vi "PhotonVision_CameraProcess.vi"(9 "Roll, Pitch, Yaw":T5, 10 "TRANSLATION3D":T2={"X"=-0.334, "Y"=0.125, "Z"=-0.22} {"Z" format="%14.3f"; "Y" format="%14.3f"; "X" format="%14.3f"}, 11 "CameraName":string="GENERAL_WEBCAM") -> (0 "out CameraToTarget_Pose3d":T1={"Translation3d"={"X"=0.0, "Y"=0.0, "Z"=0.0}, "Rotation3d"={"Q_quaternion"={"R"=1.0, "V"=[0.0, 0.0, 0.0]}}} {"Translation3d"."Z" format="%14.3f"; "Translation3d"."Y" format="%14.3f"; "Translation3d"."X" format="%14.3f"}, 1 "out RobotPose":T6 {"ROTATION"."SIN" format="%13.4f"; "ROTATION"."COS" format="%13.4f"; "ROTATION"."VALUE" format="%13.4f"; "TRANSLATION"."Y" format="%14.3f"; "TRANSLATION"."X" format="%14.3f"}, 2 "Have Multi-tag":bool, 3 "CameraName":string="GENERAL_WEBCAM", 5 "Pose Ambiguity":dbl)   [LabVIEW 2023]
uses:
  <vilib>/Rock Robotics/WPI/ThirdParty/PhotonVisionLib/PhotonVisionLib.lvlib
  <vilib>/Rock Robotics/WPI/ThirdParty/JAS_Junk/TrajLib/Trajectory_Library.lvlib
  <vilib>/Rock Robotics/Network Tables/NT Write Numeric Array.vi
  <vilib>/Rock Robotics/WPI/ThirdParty/JAS_Junk/TrajLib/TypeDef/TRANSLATION3D.ctl
  <vilib>/Rock Robotics/WPI/ThirdParty/JAS_Junk/TrajLib/TypeDef/QUATERNION.ctl
  <vilib>/Rock Robotics/WPI/ThirdParty/JAS_Junk/TrajLib/TypeDef/ROTATION3D.ctl
  <vilib>/Rock Robotics/WPI/ThirdParty/JAS_Junk/TrajLib/TypeDef/POSE3D.ctl
  <vilib>/Rock Robotics/Network Tables/NT Write Integer Array.vi
  <vilib>/Rock Robotics/Network Tables/NT Write Boolean.vi
  <vilib>/Rock Robotics/Network Tables/NT Write Integer.vi
  <vilib>/Rock Robotics/WPI/ThirdParty/JAS_Junk/TrajLib/VI/AprilTagFieldLayout_New2025.vi
  <vilib>/Rock Robotics/WPI/ThirdParty/JAS_Junk/TrajLib/TypeDef/TRANSLATION2D.ctl
  <vilib>/Rock Robotics/WPI/ThirdParty/JAS_Junk/TrajLib/TypeDef/ROTATION2D.ctl
  <vilib>/Rock Robotics/WPI/ThirdParty/JAS_Junk/TrajLib/TypeDef/POSE2D.ctl
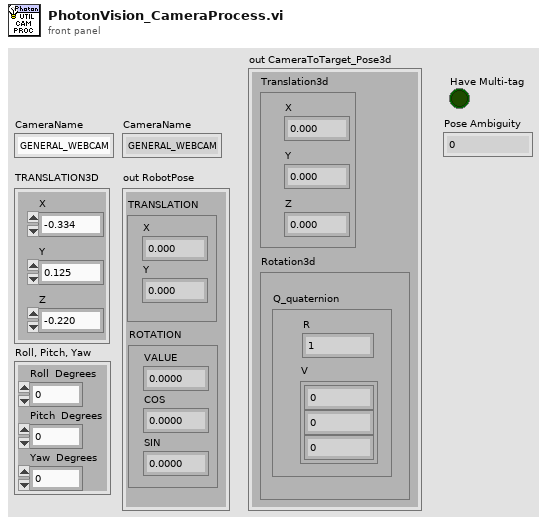
[diagram p1: front panel]
types:
  T1 = typedef "Trajectory_Library.lvlib/POSE3D.ctl" = cluster{"Translation3d":T2, "Rotation3d":T3}
  T2 = typedef "Trajectory_Library.lvlib/TRANSLATION3D.ctl" = cluster{"X":dbl, "Y":dbl, "Z":dbl}
  T3 = typedef "Trajectory_Library.lvlib/ROTATION3D.ctl" = cluster{"Q_quaternion":T4}
  T4 = typedef "Trajectory_Library.lvlib/QUATERNION.ctl" = cluster{"R":dbl, "V":dbl[]}
  T5 = cluster{"Roll  Degrees":dbl, "Pitch  Degrees":dbl, "Yaw  Degrees":dbl}
  T6 = typedef "Trajectory_Library.lvlib/POSE2D.ctl" = cluster{"TRANSLATION":T7, "ROTATION":T8}
  T7 = typedef "Trajectory_Library.lvlib/TRANSLATION2D.ctl" = cluster{"X":dbl, "Y":dbl}
  T8 = typedef "Trajectory_Library.lvlib/ROTATION2D.ctl" = cluster{"VALUE":dbl, "COS":dbl, "SIN":dbl}
  T9 = typedef "PhotonVisionLib.lvlib/PhotonPipelineResultType.ctl" = cluster{"TargetCount":i32, "Latency_MilliSec":dbl, "Targets":T10[], "TimeStampSec":dbl, "PhotonMultiTargetPNPResult":T13}
  T10 = typedef "PhotonVisionLib.lvlib/PhotonTrackedTargetType.ctl" = cluster{"Yaw":dbl, "Pitch":dbl, "Area":dbl, "Skew":dbl, "MinAreaRectCorners":T11[], "BestCameraToTarget":T12, "FiiducialId":i32, "AltCameraToTarget":T12, "PoseAmbiguity":dbl, "DetectedCorners":T11[]}
  T11 = typedef "PhotonVisionLib.lvlib/TargetCornerType.ctl" = cluster{"X":dbl, "Y":dbl}
  T12 = typedef "Trajectory_Library.lvlib/TRANSFORM3D.ctl" = cluster{"TRANSLATION3D":T2, "ROTATION3D":T3, "XF":bool}
  T13 = typedef "PhotonVisionLib.lvlib/PhotonMultiTargetPNPResultType.ctl" = cluster{"PhotonPNPResult":T14, "FiducialIDsUsed":i16[]}
  T14 = typedef "PhotonVisionLib.lvlib/PhotonPNPResultType.ctl" = cluster{"IsPresent":bool, "bestReprojErr":dbl, "altReprojErr":dbl, "ambiguity":dbl, "Best":T12, "Alt":T12}
  T15 = typedef "Trajectory_Library.lvlib/AprilTagFieldLayout.ctl" = cluster{"AprilTagMap":map{i32, T16}, "FieldLength":dbl, "FieldWidth":dbl, "OriginPosition ":T17, "OriginPose3d":T1}
  T16 = typedef "Trajectory_Library.lvlib/AprilTag.ctl" = cluster{"ID":i32, "POSE3D":T1}
  T17 = typedef "Trajectory_Library.lvlib/AprilTagFieldLayoutOrignPosition_ENUM.ctl" = enum16{"kBlueAllianceWallRightSide,", "kRedAllianceWallRightSide,"}
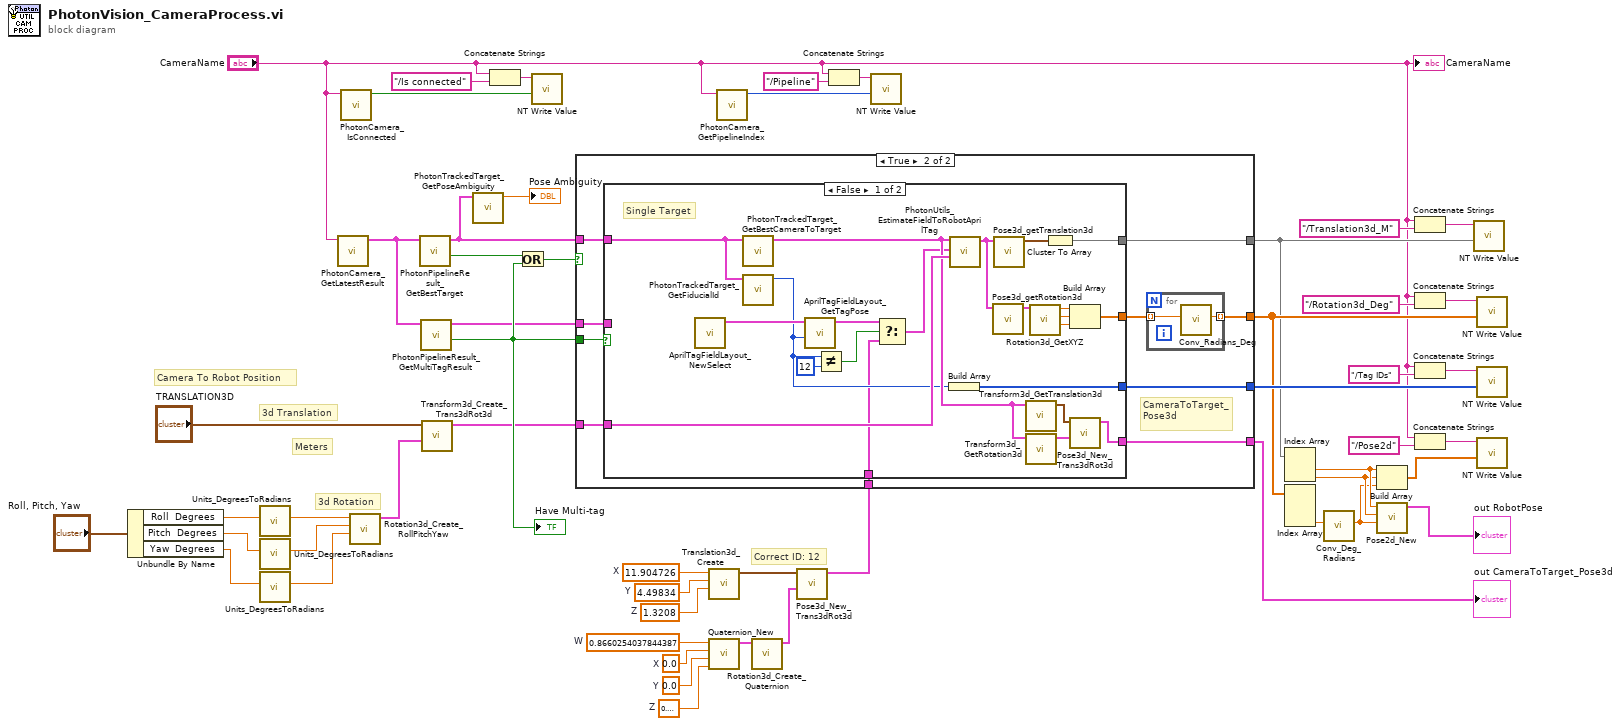
[diagram p0: block diagram]
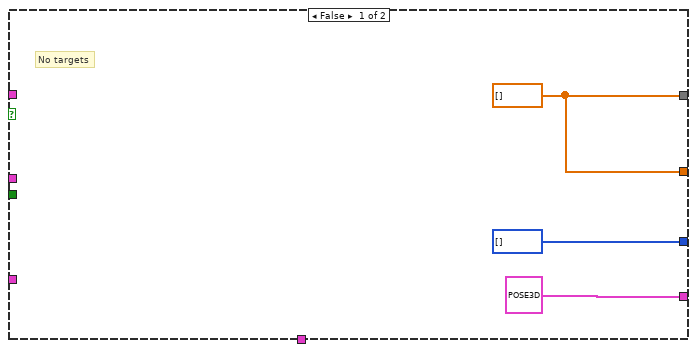
[diagram p2: hidden frame]
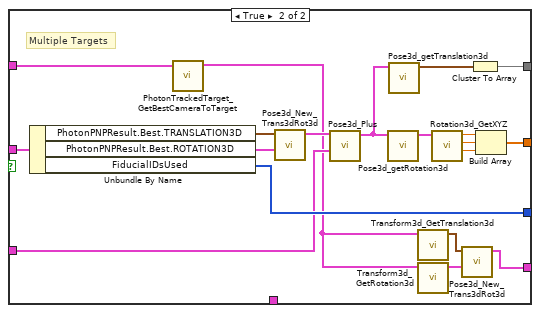
[diagram p3: hidden frame]
diagram:
  w3 = 11.904726  # X
  w4 = 4.49834  # Y
  w5 = 1.3208  # Z
  w2 = 0.8660254037844387  # W
  w6 = 0.0  # X
  w7 = 0.0  # Y
  w8 = 0.49999999999999994  # Z
  # "Correct ID: 12"
  # "Meters"
  # "Camera To Robot Position"
  # "3d Rotation"
  # "3d Translation"
  n1 = Unbundle By Name("Roll, Pitch, Yaw") -> ("Roll  Degrees"=w19:dbl, "Pitch  Degrees"=w18:dbl, "Yaw  Degrees"=w17:dbl)
  n2 = call <vilib>:"Units_DegreesToRadians.vi"("Degrees"=w19) -> ("Radians"=w46:dbl)  [unwired: 10 in]
  n3 = call <vilib>:"Units_DegreesToRadians.vi"("Degrees"=w18) -> ("Radians"=w45:dbl)  [unwired: 10 in]
  n4 = call <vilib>:"Units_DegreesToRadians.vi"("Degrees"=w17) -> ("Radians"=w44:dbl)  [unwired: 10 in]
  n5 = call <vilib>:"PhotonCamera_GetLatestResult.vi"("CameraName"="CameraName") -> ("PipelineResult"=w52:T9)  [unwired: 7 in, 3 out]
  n6 = call <vilib>:"PhotonCamera_IsConnected.vi"("CameraName"="CameraName") -> ("IsConnected"=w53:bool)  [unwired: 9 in, 1 out]
  n7 = call <vilib>:"Rotation3d_Create_RollPitchYaw.vi"("Yaw"=w44, "Pitch"=w45, "Roll"=w46) -> ("Rotation3d"=w47:T3)  [unwired: 8 in]
  n8 = call <vilib>:"PhotonPipelineResult_GetBestTarget.vi"("PhotonPipelineResult"=w52) -> ("TargetFound"=w51:bool, "PhotonTrackedTarget"=w13:T10)  [unwired: 9 in]
  n9 = call <vilib>:"PhotonPipelineResult_GetMultiTagResult.vi"("PhotonPipelineResult"=w52) -> ("Is Present"=w49:bool, "PhotonMultiTargetPNPResult"=w48:T13)  [unwired: 9 in]
  "Have Multi-tag" <- w49
  n10 = call <vilib>:"Transform3d_Create_Trans3dRot3d.vi"("Rotation3d"=w47, "Translation3d"="TRANSLATION3D") -> ("Transform3d"=w43:T12)  [unwired: 9 in]
  n11 = call <vilib>:"PhotonTrackedTarget_GetPoseAmbiguity.vi"("TrackedTarget"=w13) -> ("Pose Ambiguity"=→"Pose Ambiguity":dbl)  [unwired: 10 in]
  n12 = Concatenate Strings("CameraName", "/Is connected" ("name")) -> (w40:string)
  n13 = Or(x=w51, y=w49) -> (x .or. y?=w50:bool)
  n14 = call-poly <vilib>:"NT Write Value.vi"("value"=w53, "name"=w40) -> ()  [unwired: 9 in, 1 out]
  n15 = call <vilib>:"Translation3d_Create.vi"("Z"=w5, "Y"=w4, "X"=w3) -> ("TRANSLATION3D"=w11:T2)  [unwired: 8 in]
  n16 = call <vilib>:"Quaternion_New.vi"("Z"=w8, "Y"=w7, "X"=w6, "W"=w2) -> ("out Quaternion"=w9:T4)  [unwired: 7 in]
  n17 = call <vilib>:"PhotonCamera_GetPipelineIndex.vi"("CameraName"="CameraName") -> ("PipelineIndex"=w25:i32)  [unwired: 9 in, 1 out]
  n18 = call <vilib>:"Rotation3d_Create_Quaternion.vi"("Quaternion"=w9) -> ("Rotation3d"=w10:T3)  [unwired: 10 in]
  n19 = call <vilib>:"Pose3d_New_Trans3dRot3d.vi"("Rotation3d"=w10, "Translation3d"=w11) -> ("outPose3d"=w1:T1)  [unwired: 9 in]
  n20 = case shown="True" w50 {
    tunnel: w49 -> [_ w66]
    tunnel: w13 -> [_ w65]
    tunnel: w48 -> [_ w64]
    tunnel: w43 -> [_ w63]
    tunnel: [w56 w62] -> w29
    tunnel: [w56 w59] -> w31
    tunnel: [i16[] [] ("FiducialIDsUsed") w61] -> w42
    tunnel: [T1 {"Translation3d"={"X"=0.0, "Y"=0.0, "Z"=0.0}, "Rotation3d"={"Q_quaternion"={"R"=1.0, "V"=[0.0, 0.0, 0.0]}}} ("outPose3d") w58] -> w14
    tunnel: w1 -> [_ w57]
    frame False {
      w56 = dbl[] [] ("out Translation3d")
      # "No targets"
    }
    frame True {
      # "CameraToTarget_Pose3d"
      n21 = case shown="False" w66 {
        tunnel: w65 -> [w90 w95]
        tunnel: w64 -> [_ w109]
        tunnel: w63 -> [w88 w102]
        tunnel: [w81 w98] -> w62
        tunnel: [w80 w105] -> w61
        tunnel: [w79 w97] -> w60
        tunnel: [w75 w91] -> w58
        tunnel: w57 -> [w69 _]
        frame False {
          # "Single Target"
          n22 = call-poly <vilib>:"AprilTagFieldLayout_NewSelect.vi"() -> ("AprilTagFieldLayout"=w89:T15)  [unwired: 11 in]
          n23 = call <vilib>:"PhotonTrackedTarget_GetBestCameraToTarget.vi"("TrackedTarget"=w90) -> ("BestCameraToTarget"=w76:T12)  [unwired: 9 in, 1 out]
          n24 = call <vilib>:"PhotonTrackedTarget_GetFiducialId.vi"("TrackedTarget"=w90) -> ("Fiducial Id"=w74:i32)  [unwired: 10 in]
          n25 = call <vilib>:"AprilTagFieldLayout_GetTagPose.vi"("TagId"=w74, "AprilTagFieldLayout"=w89) -> ("TagPose3d"=w71:T1)  [unwired: 8 in, 1 out]
          n26 = Not Equal?(x=w74, y=12) -> (x != y?=w72:bool)
          n27 = Select(t=w71, s=w72, f=w69) -> (s? t:f=w70:T1)
          n28 = Build Array(w74) -> (w80:i32[])
          n29 = call <vilib>:"PhotonUtils_EstimateFieldToRobotAprilTag.vi"("CameraToRobotTransform3d"=w88, "FieldRelativeTagPose3d"=w70, "CameraToTargetTransform3d"=w76) -> ("FieldToRpbotPose3d"=w87:T1)  [unwired: 8 in]
          n30 = call <vilib>:"Pose3d_getRotation3d.vi"("in Pose3d"=w87) -> ("out Rotation3d"=w86:T3)  [unwired: 10 in]
          n31 = call <vilib>:"Pose3d_getTranslation3d.vi"("in Pose3d"=w87) -> ("out Translation3d"=w82:T2)  [unwired: 10 in]
          n32 = call <vilib>:"Transform3d_GetTranslation3d.vi"("in Transform3d"=w76) -> ("Translation3d"=w78:T2)  [unwired: 10 in]
          n33 = call <vilib>:"Transform3d_GetRotation3d.vi"("in Transform3d"=w76) -> ("Rotation3d"=w77:T3)  [unwired: 10 in]
          n34 = call <vilib>:"Rotation3d_GetXYZ.vi"("in Rotation3d"=w86) -> ("Z"=w83:dbl, "Y"=w84:dbl, "X"=w85:dbl)  [unwired: 8 in]
          n35 = Cluster To Array(cluster=w82) -> (array=w81:dbl[])
          n36 = Build Array(w85, w84, w83) -> (w79:dbl[])
          n37 = call <vilib>:"Pose3d_New_Trans3dRot3d.vi"("Rotation3d"=w77, "Translation3d"=w78) -> ("outPose3d"=w75:T1)  [unwired: 9 in]
        }
        frame True {
          # "Multiple Targets"
          n38 = Unbundle By Name(w109) -> ("PhotonPNPResult.Best.TRANSLATION3D"=w104:T2, "PhotonPNPResult.Best.ROTATION3D"=w103:T3, "FiducialIDsUsed"=w105:i16[])
          n39 = call <vilib>:"PhotonTrackedTarget_GetBestCameraToTarget.vi"("TrackedTarget"=w95) -> ("BestCameraToTarget"=w92:T12)  [unwired: 9 in, 1 out]
          n40 = call <vilib>:"Pose3d_New_Trans3dRot3d.vi"("Rotation3d"=w103, "Translation3d"=w104) -> ("outPose3d"=w96:T1)  [unwired: 9 in]
          n41 = call <vilib>:"Pose3d_Plus.vi"("other Transform3d"=w102, "in Pose3d"=w96) -> ("out Pose3d"=w100:T1)  [unwired: 9 in]
          n42 = call <vilib>:"Pose3d_getRotation3d.vi"("in Pose3d"=w100) -> ("out Rotation3d"=w101:T3)  [unwired: 10 in]
          n43 = call <vilib>:"Pose3d_getTranslation3d.vi"("in Pose3d"=w100) -> ("out Translation3d"=w99:T2)  [unwired: 10 in]
          n44 = call <vilib>:"Transform3d_GetTranslation3d.vi"("in Transform3d"=w92) -> ("Translation3d"=w94:T2)  [unwired: 10 in]
          n45 = call <vilib>:"Transform3d_GetRotation3d.vi"("in Transform3d"=w92) -> ("Rotation3d"=w93:T3)  [unwired: 10 in]
          n46 = call <vilib>:"Rotation3d_GetXYZ.vi"("in Rotation3d"=w101) -> ("Z"=w106:dbl, "Y"=w107:dbl, "X"=w108:dbl)  [unwired: 8 in]
          n47 = call <vilib>:"Pose3d_New_Trans3dRot3d.vi"("Rotation3d"=w93, "Translation3d"=w94) -> ("outPose3d"=w91:T1)  [unwired: 9 in]
          n48 = Cluster To Array(cluster=w99) -> (array=w98:dbl[])
          n49 = Build Array(w108, w107, w106) -> (w97:dbl[])
        }
      }
      n50 = for {
        tunnel: w60 -> [w68] mode=indexing
        tunnel: [w67] -> w59 mode=indexing
        n51 = call <vilib>:"Conv_Radians_Deg.vi"("Radians"=w68) -> ("Degrees"=w67:dbl)  [unwired: 10 in]
      }
    }
  }
  "out CameraToTarget_Pose3d" <- w14
  n52 = Concatenate Strings("CameraName", "/Pipeline" ("name")) -> (w27:string)
  n53 = call-poly <vilib>:"NT Write Value.vi"("value"=w25, "name"=w27) -> ()  [unwired: 9 in, 1 out]
  n54 = Index Array(array=w29) -> (element #1=w24:dbl, element #2=w23:dbl)  [unwired: 2 in]
  n55 = Index Array(array=w31) -> (element #3=w30:dbl)  [unwired: 3 in, 2 out]
  n56 = call <vilib>:"Conv_Deg_Radians.vi"("Degress"=w30) -> ("Radians"=w15:dbl)  [unwired: 10 in]
  n57 = Build Array(w24, w23, w15) -> (w28:dbl[])
  n58 = call <vilib>:"Pose2d_New.vi"("Heading"=w15, "Y"=w23, "X"=w24) -> ("out POSe"=→"out RobotPose":T6)  [unwired: 8 in]
  n59 = Concatenate Strings("CameraName", "/Translation3d_M" ("name")) -> (w38:string)
  n60 = Concatenate Strings("CameraName", "/Rotation3d_Deg" ("name")) -> (w36:string)
  n61 = Concatenate Strings("CameraName", "/Tag IDs" ("name")) -> (w34:string)
  n62 = Concatenate Strings("CameraName", "/Pose2d" ("name")) -> (w33:string)
  n63 = call-poly <vilib>:"NT Write Value.vi"("value"=w29, "name"=w38) -> ()  [unwired: 9 in, 1 out]
  n64 = call-poly <vilib>:"NT Write Value.vi"("value"=w31, "name"=w36) -> ()  [unwired: 9 in, 1 out]
  n65 = call-poly <vilib>:"NT Write Value.vi"("value"=w42, "name"=w34) -> ()  [unwired: 9 in, 1 out]
  n66 = call-poly <vilib>:"NT Write Value.vi"("value"=w28, "name"=w33) -> ()  [unwired: 9 in, 1 out]
  "CameraName" <- "CameraName"
